vi "Read_FFID_Auto_Calib_Setup.vi"(5 "Specific Argument":string) -> (0 "Trace concentration %":dbl[](array[numeric]), 1 "Carrier 2 Q":dbl[](array[numeric]), 2 "Carrier 1 Q":dbl[](array[numeric]), 3 "Mix_own_Calib_Gases":bool, 4 "Error String":string)   [LabVIEW 2014]
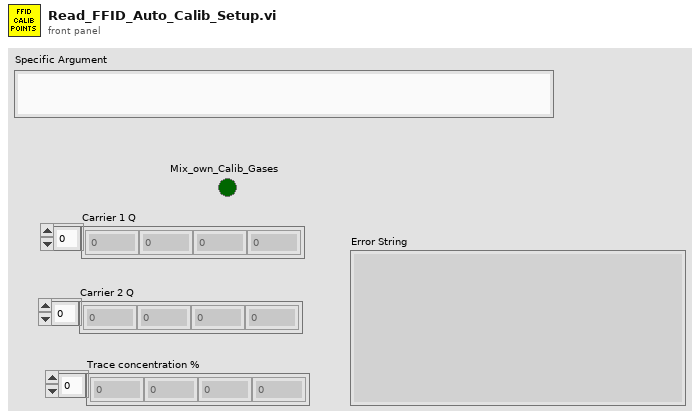
[diagram p1: front panel]
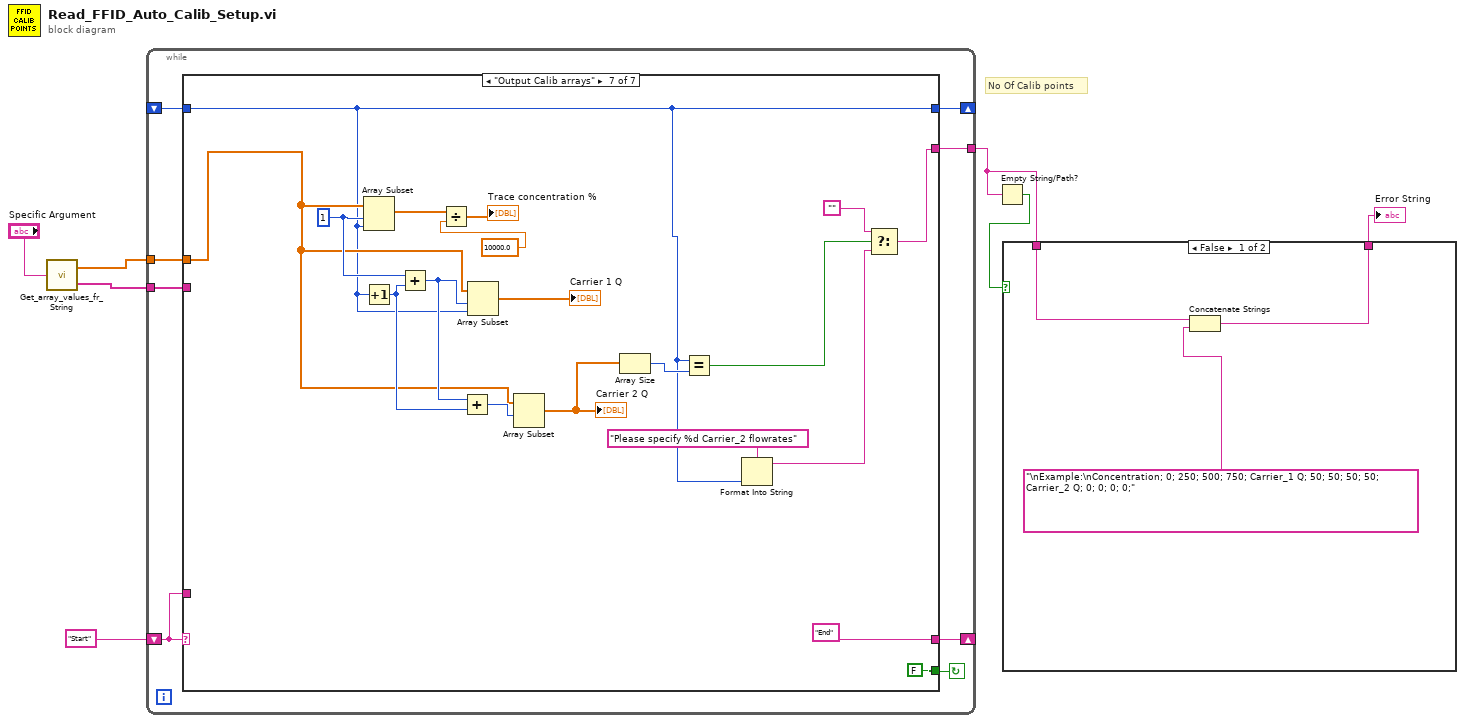
[diagram p0: block diagram]
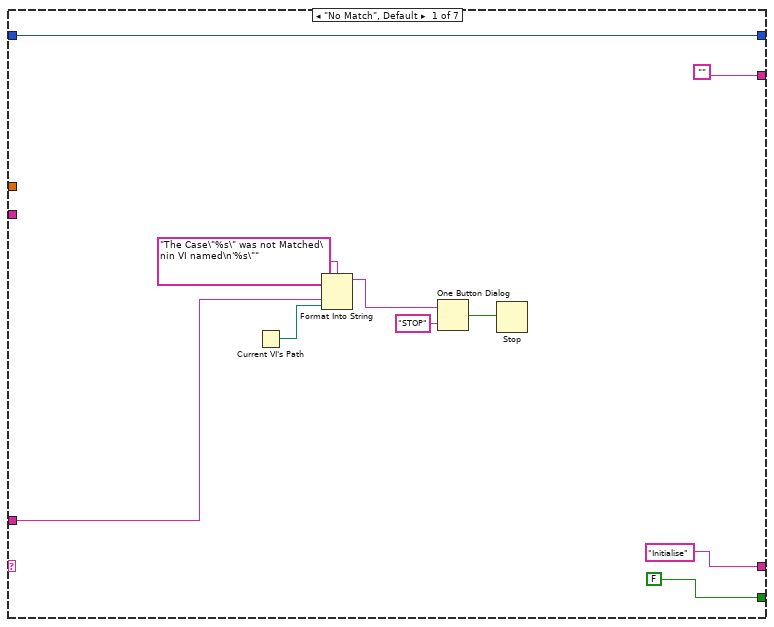
[diagram p3: hidden frame]
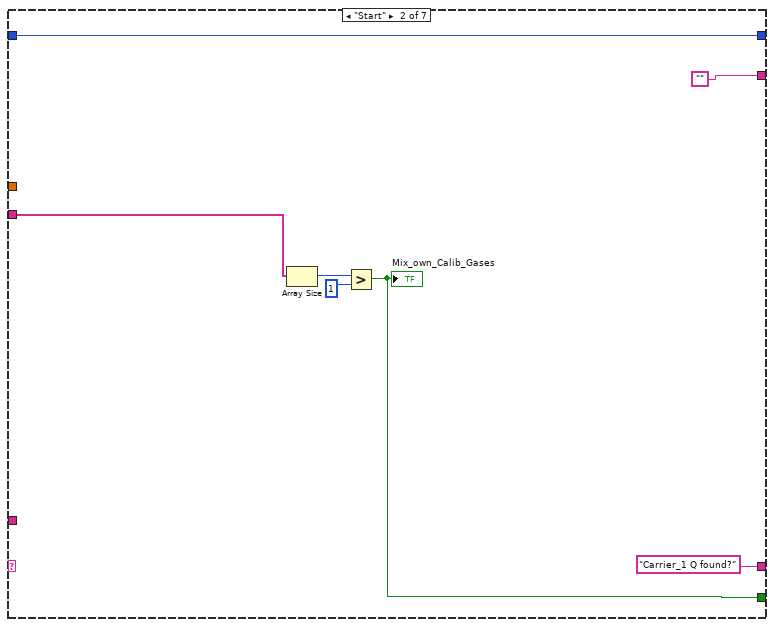
[diagram p4: hidden frame]
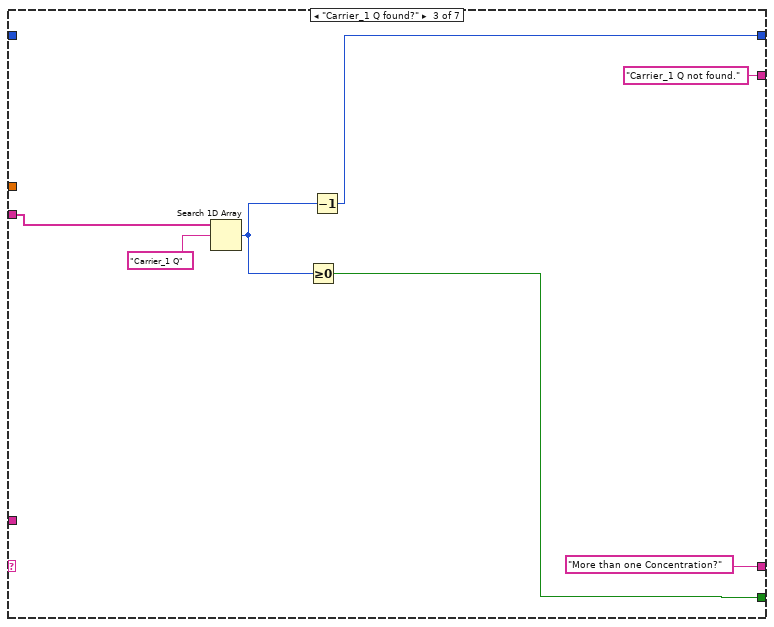
[diagram p5: hidden frame]
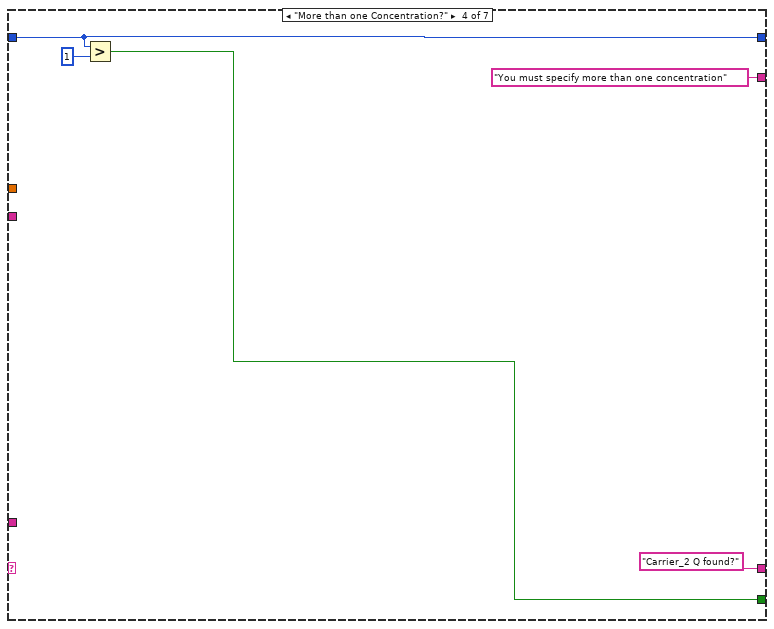
[diagram p6: hidden frame]
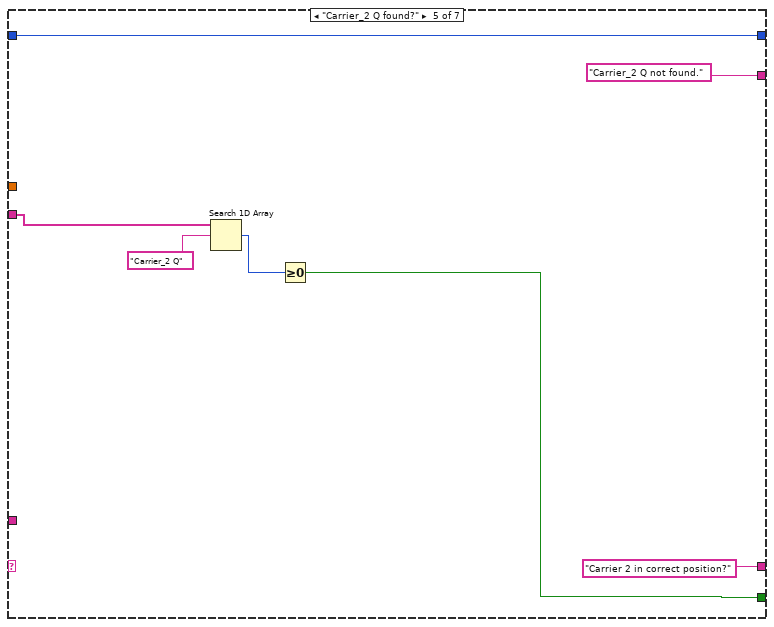
[diagram p7: hidden frame]
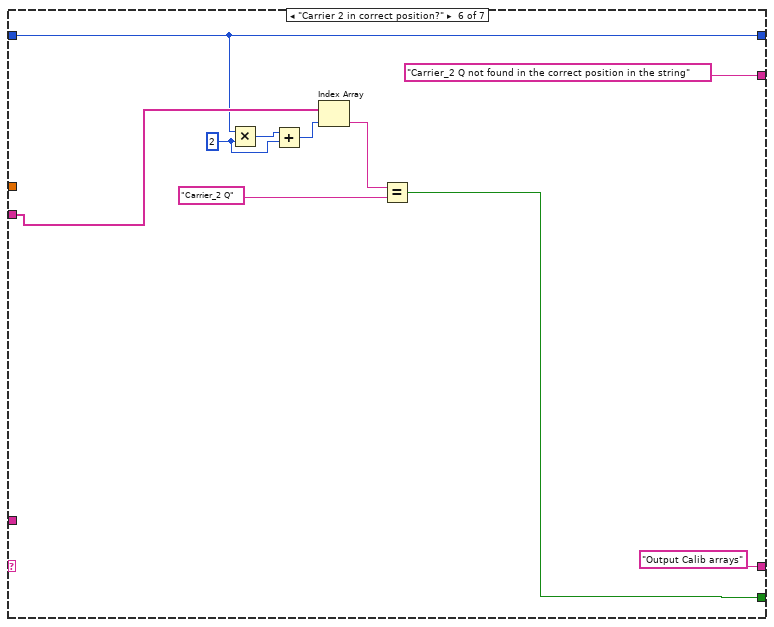
[diagram p8: hidden frame]
diagram:
  # "No Of Calib points"
  n1 = call "Get_array_values_fr_String.vi"("String Value"="Specific Argument") -> ("Numeric Array"=w4:dbl[], "String array"=w5:string[])
  n2 = while {
    shift-left: "Start" -> [w13]
    shift-right: [w14] -> _
    tunnel: w5 -> [w12]
    tunnel: [w11] -> w1
    shift-right: [w10] -> _
    shift-left: _ -> [w9]
    tunnel: w4 -> [w8]
    stop <- w15 continue-if-true
    n3 = case shown="\"Output Calib arrays\"" w13 {
      tunnel: [FALSE w28 w36 w40 w45 w57 FALSE] -> w15
      tunnel: ["Initialise" "Carrier_1 Q found?" "More than one Concentration?" "Carrier_2 Q found?" "Carrier 2 in correct position?" "Output Calib arrays" "End"] -> w14
      tunnel: w13 -> [w20 _ _ _ _ _ _]
      tunnel: w12 -> [_ w29 w37 _ w49 w60 _]
      tunnel: ["" "" "Carrier_1 Q not found." "You must specify more than one concentration" "Carrier_2 Q not found." "Carrier_2 Q not found in the correct position in the string" w66] -> w11
      tunnel: [w17 w26 w33 w41 w48 w59 w64] -> w10
      tunnel: w9 -> [w17 w26 _ w41 w48 w59 w64]
      tunnel: w8 -> [_ _ _ _ _ _ w75]
      frame "No Match", Default {
        n4 = Current VI's Path() -> (path=w19:path)
        n5 = Format Into String(format string="The Case\"%s\" was not Matched\nin VI named\n'%s\"" ("Format String"), w20, w19) -> (resulting string=w23:string)  [unwired: 2 in, 1 out]
        n6 = One Button Dialog(message=w23, button name ("OK")="STOP") -> (true=w21:bool)
        n7 = Stop(stop? (T)=w21) -> ()
      }
      frame "Start" {
        n8 = Array Size(array=w29) -> (size(s)=w31:i32)
        n9 = Greater?(x=w31, y=1) -> (0:w28:bool)
        "Mix_own_Calib_Gases" <- w28
      }
      frame "Carrier_1 Q found?" {
        n10 = Search 1D Array(1D array=w37, element="Carrier_1 Q") -> (index of element=w34:i32)  [unwired: 1 in]
        n11 = Greater Or Equal To 0?(x=w34) -> (x >= 0?=w36:bool)
        n12 = Decrement(x=w34) -> (x-1=w33:i32)
      }
      frame "More than one Concentration?" {
        n13 = Greater?(x=w41, y=1) -> (0:w40:bool)
      }
      frame "Carrier_2 Q found?" {
        n14 = Search 1D Array(1D array=w49, element="Carrier_2 Q") -> (index of element=w50:i32)  [unwired: 1 in]
        n15 = Greater Or Equal To 0?(x=w50) -> (x >= 0?=w45:bool)
      }
      frame "Carrier 2 in correct position?" {
        w53 = 2 ("y")
        n16 = Multiply(x=w59, y=w53) -> (x*y=w54:i32)
        n17 = Add(x=w54, y=w53) -> (x+y=w52:i32)
        n18 = Index Array(array=w60, index=w52) -> (element=w58:string)
        n19 = Equal?(x=w58, y="Carrier_2 Q" ("element")) -> (x = y?=w57:bool)
      }
      frame "Output Calib arrays" {
        w79 = 1 ("index")
        n20 = Array Subset(array=w75, index=w79, length=w64) -> (w74:dbl[])
        n21 = Increment(x=w64) -> (x+1=w77:i32)
        n22 = Add(x=w79, y=w77) -> (x+y=w78:i32)
        n23 = Divide(x=w74, y=10000.0) -> (x/y=→"Trace concentration %":dbl[])
        n24 = Add(x=w78, y=w77) -> (x+y=w76:i32)
        n25 = Array Subset(array=w75, index=w78, length=w64) -> (→"Carrier 1 Q":dbl[])
        n26 = Array Subset(array=w75, index=w76) -> (w71:dbl[])  [unwired: 1 in]
        "Carrier 2 Q" <- w71
        n27 = Array Size(array=w71) -> (size(s)=w68:i32)
        n28 = Equal?(x=w64, y=w68) -> (x = y?=w65:bool)
        n29 = Format Into String(format string="Please specify %d Carrier_2 flowrates", w64) -> (resulting string=w62:string)  [unwired: 2 in, 1 out]
        n30 = Select(t="", s=w65, f=w62) -> (s? t:f=w66:string)
      }
    }
  }
  n31 = Empty String/Path?(string/path=w1) -> (empty?=w3:bool)
  n32 = case shown="False" w3 {
    tunnel: [w81 w84] -> w2
    tunnel: w1 -> [w82 w84]
    frame False {
      n33 = Concatenate Strings(w82, "\nExample:\nConcentration; 0; 250; 500; 750; Carrier_1 Q; 50; 50; 50; 50; Carrier_2 Q; 0; 0; 0; 0;") -> (w81:string)
    }
    frame True {
    }
  }
  "Error String" <- w2
